vi "zslower.vi"(9 "maxvel":dbl, 10 "labview_zpos_write":dbl, 11 "nanonis_zpos_read":dbl) -> (3 "function return":dbl)   [LabVIEW 2017, in "HapticSTM.lvlib"]
doc: "extern \"C\" __declspec(dllexport) double zslower(double nanonis_zpos_read, double labview_zpos_write, double maxvel);"
uses:
  <userlib>/HapticSTM/Feedbackless - Testdata/HapticSTM.lvlib
  <userlib>/HapticSTM/HapticSTM.dll
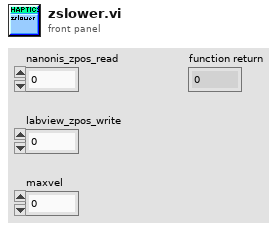
[diagram p1: front panel]
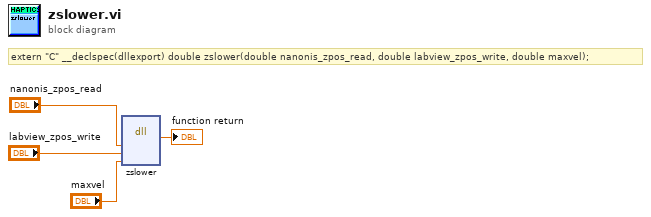
[diagram p0: block diagram]
diagram:
  # "extern \"C\" __declspec(dllexport) double zslower(double nanonis_zpos_read, double labview_zpos_write, double maxvel);"
  n1 = dll-call lib="C:/Program Files/National Instruments/LabVIEW 2019/user.lib/HapticSTM/HapticSTM.*" fn="zslower"("nanonis_zpos_read"="nanonis_zpos_read", "labview_zpos_write"="labview_zpos_write", "maxvel"="maxvel") -> (→"function return":dbl)  [unwired: 6 in, 2 out]
